vi "Split TargetPanel by Node.vi"(8 "error in":errorcluster caption="错误输入（无错误）", 9 "Split Mode":T1, 10 "Node*":refnum<data-value>, 11 "PanelRootNode 输入":refnum<class "PanelRootNode.lvclass"> caption="DNL_LabVIEW Object in") -> (0 "error out":errorcluster caption="错误输出", 2 "ChildDataNode[]":refnum<data-value>[](array[refnum]), 3 "PanelRootNode 输出":refnum<class "PanelRootNode.lvclass"> caption="DNL_LabVIEW Object out")   [LabVIEW 2013, in "PanelRootNode.lvclass"]
uses:
  PanelRootNode.lvclass
  PanelObject/PanelObject.lvclass
  PanelDataNode/Split Mode.ctl
  PanelDataNode/PanelDataNode.lvclass
  PanelLinkNode/PanelLinkNode.lvclass/PanelLinkNode.ctl
  PanelLinkNode/PanelLinkNode.lvclass
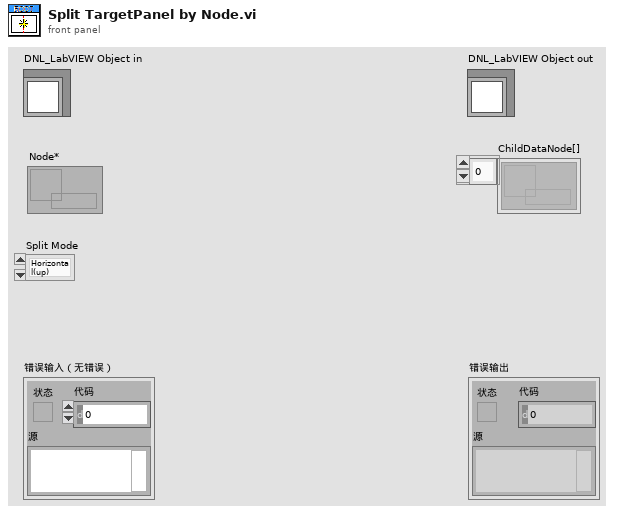
[diagram p1: front panel]
types:
  T1 = typedef "PanelDataNode.lvclass/Split Mode.ctl" = enum16{"Horizontal(up)", "Vertical(left)", "Horizontal(down)", "Vertical(right)"}
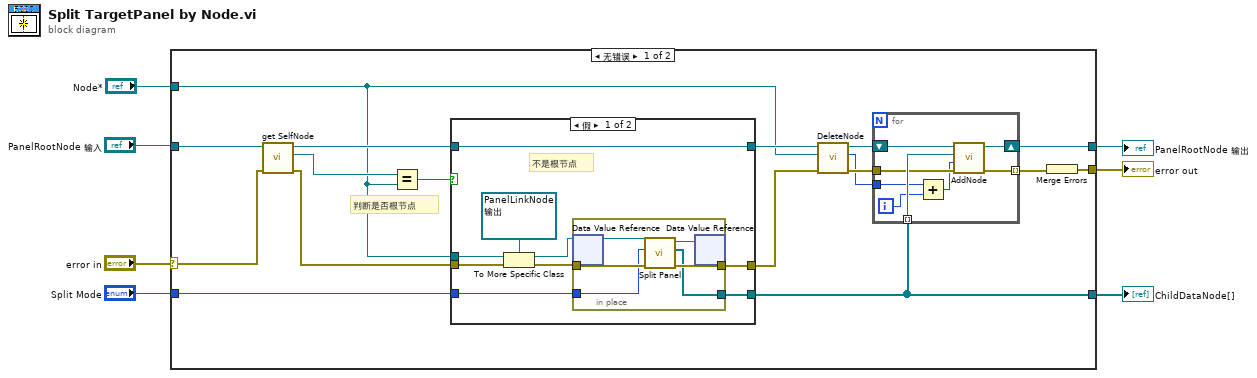
[diagram p0: block diagram]
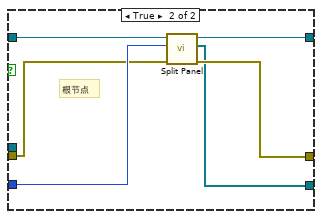
[diagram p2: hidden frame]
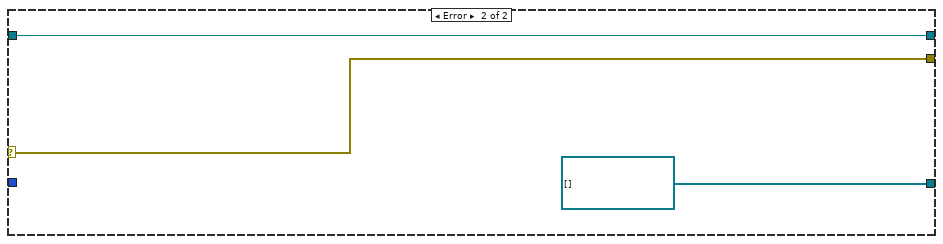
[diagram p3: hidden frame]
diagram:
  n1 = case shown="无错误" "error in" {
    selector: "error in" -> [w16 w56]
    tunnel: [w9 w56] -> w3
    tunnel: [w13 w55] -> w7
    tunnel: "PanelRootNode 输入" -> [w20 w55]
    tunnel: "Node*" -> [w15 _]
    tunnel: "Split Mode" -> [w21 _]
    tunnel: [w12 refnum<data-value>[] [] ("ChildDataNode[]")] -> w1
    frame No Error {
      # "判断是否根节点"
      n2 = call "get SelfNode.vi"("error in (no error)"=w16, "PanelLinkNode输入"=w20) -> ("error out"=w17:errorcluster, "SelfNode*"=w23:refnum<data-value>, "PanelLinkNode输出"=w24:refnum<class "PanelRootNode.lvclass">)  [unwired: 7 in]
      n3 = Equal?(x=w23, y=w15) -> (x = y?=w22:bool)
      n4 = case shown="假" w22 {
        tunnel: [w41 w53] -> w18
        tunnel: w24 -> [w40 w52]
        tunnel: [w40 w51] -> w19
        tunnel: w15 -> [w37 _]
        tunnel: w21 -> [w35 w50]
        tunnel: [w34 w49] -> w12
        tunnel: w17 -> [w33 w48]
        frame False {
          # "不是根节点"
          n5 = To More Specific Class(target class=refnum<data-value> refnum ("数据值引用"), reference=w37, error in=w33) -> (specific class reference=w39:refnum<data-value>, error out=w38:errorcluster)
          n6 = in-place {
            in-place-border: w38 -> [w44]
            in-place-border: [w45] -> w41
            in-place-border: w35 -> [w43]
            in-place-border: [w42] -> w34
            n7 = in-place-dvr #1(w39) -> (w47:refnum<class "PanelRootNode.lvclass">)  [unwired: 1 out]
            n8 = call-dynamic "Split Panel.vi"("error in (no error)"=w44, "Split Mode"=w43, "PanelDataNode 输入"=w47) -> ("error out"=w45:errorcluster, "ChildDataNode[]"=w42:refnum<data-value>[], "PanelDataNode 输出"=w46:refnum<class "PanelRootNode.lvclass">)  [unwired: 6 in]
            n9 = in-place-dvr #1(w46) -> ()  [unwired: 2 out]
          }
        }
        frame True {
          # "根节点"
          n10 = call-dynamic "Split Panel.vi"("error in (no error)"=w48, "Split Mode"=w50, "PanelDataNode 输入"=w52) -> ("error out"=w53:errorcluster, "ChildDataNode[]"=w49:refnum<data-value>[], "PanelDataNode 输出"=w51:refnum<class "PanelRootNode.lvclass">)  [unwired: 6 in]
        }
      }
      n11 = call "DeleteNode.vi"("error in (no error)"=w18, "Node*"=w15, "PanelRootNode 输入"=w19) -> ("error out"=w11:errorcluster, "index"=w8:i32, "PanelRootNode 输出"=w14:refnum<class "PanelRootNode.lvclass">)  [unwired: 6 in]
      n12 = for {
        tunnel: w12 -> [w30] mode=indexing
        tunnel: w11 -> [w29]
        shift-right: [w31] -> w13
        shift-left: w14 -> [w32]
        tunnel: [w28] -> w10 mode=indexing
        tunnel: w8 -> [w27]
        i -> [w26]
        n13 = Add(x=w27, y=w26) -> (x+y=w25:i32)
        n14 = call "AddNode.vi"("error in (no error)"=w29, "Index"=w25, "Node*"=w30, "PanelRootNode 输入"=w32) -> ("error out"=w28:errorcluster, "PanelRootNode 输出"=w31:refnum<class "PanelRootNode.lvclass">)  [unwired: 6 in]
      }
      n15 = Merge Errors(w10) -> (w9:errorcluster)
    }
    frame Error {
    }
  }
  "error out" <- w3
  "PanelRootNode 输出" <- w7
  "ChildDataNode[]" <- w1
